vi "Update Version.vi"(8 "error in (no error)":errorcluster, 11 "GitPackage in":refnum<class "GitPackage.lvclass">) -> (0 "error out":errorcluster, 3 "GitPackage out":refnum<class "GitPackage.lvclass">)   [LabVIEW 2020, in "GPack.lvlib" / "GitPackage.lvclass"]
uses:
  GitPackage.lvclass
  GitPackage.lvclass/GitPackage.ctl
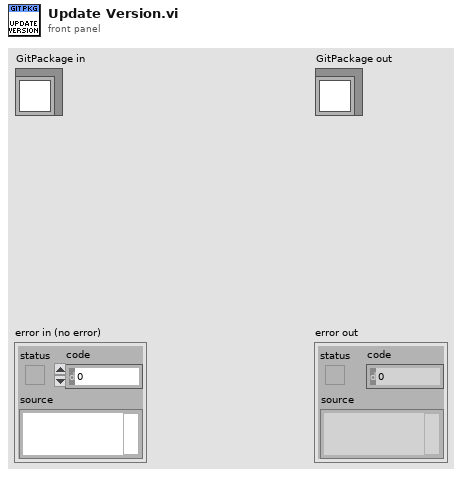
[diagram p1: front panel]
types:
  T1 = typedef "GPack.lvlib/Package Info.ctl" = cluster{"Name":string, "Type":string, "Host":string, "Path":string, "Branch":string, "Version":string, "License":string}
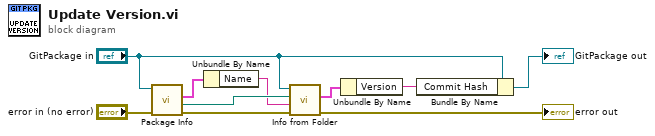
[diagram p0: block diagram]
diagram:
  n1 = call-dynamic "Package Info.vi"("error in (no error)"="error in (no error)", "GitPackage in"="GitPackage in") -> ("error out"=w8:errorcluster, "Folder"=w9:path, "Package Info"=w7:T1)  [unwired: 7 in]
  n2 = Unbundle By Name(w7) -> ("Name"=w6:string)
  n3 = call-dynamic "Info from Folder.vi"("error in (no error)"=w8, "Name"=w6, "Folder"=w9, "GitPackage in"="GitPackage in") -> ("error out"=→"error out":errorcluster, "Package Info"=w4:T1)  [unwired: 6 in]
  n4 = Unbundle By Name(w4) -> ("Version"=w3:string)
  n5 = Bundle By Name(cluster="GitPackage in", "Commit Hash"=w3) -> (→"GitPackage out":refnum<class "GitPackage.lvclass">)
